vi "constructor.vi"(8 "error in (no error)":errorcluster, 9 "deviceDataBase":refnum<class "deviceDataBase.lvclass">, 10 "Path":path, 11 "compiledTime":timestamp) -> (0 "error out":errorcluster, 1 "error":bool, 2 "DeviceArray":refnum<class "DeviceArray.lvclass">, 3 "ScriptListCompiler out":refnum<class "ScriptListCompiler.lvclass">)   [LabVIEW 2009, in "Compiler.lvlib" / "ScriptListCompiler.lvclass"]
uses:
  ScriptListCompiler.lvclass
  DatabaseHelpers/DbConnection/DeviceDataBase/deviceDataBase.lvclass
  DatabaseHelpers/Database Objects/DeviceArray/DeviceArray.lvclass
  Scripting/DataPointScript/DataPointScript.lvclass
  ScriptListCompiler.lvclass/ScriptListCompiler.ctl
  Scripting/ScriptingEvent/ScriptEventList/ScriptEventList.lvclass
  Compiler.lvlib
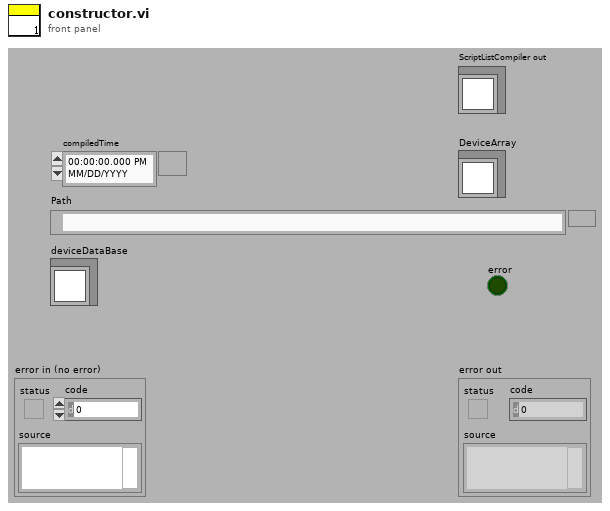
[diagram p1: front panel]
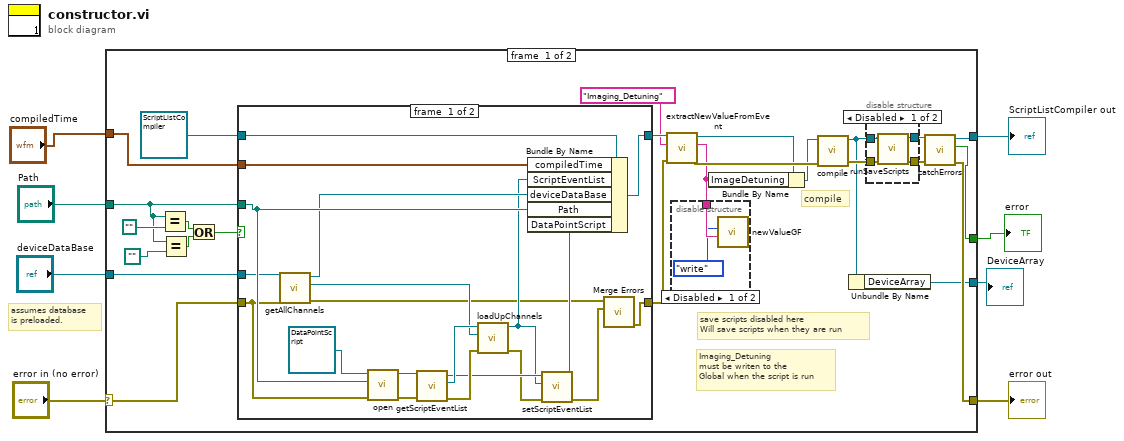
[diagram p0: block diagram]
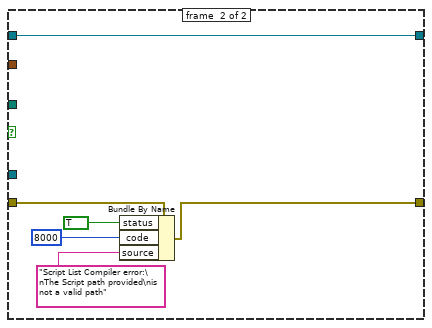
[diagram p4: hidden frame]
diagram:
  # "assumes database\nis preloaded."
  n1 = case shown="No Error" "error in (no error)" {
    selector: "error in (no error)" -> [w25 w68]
    tunnel: [w23 w68] -> w7
    tunnel: [w24 _] -> w4
    tunnel: "Path" -> [w26 _]
    tunnel: "deviceDataBase" -> [w29 _]
    tunnel: [w22 _] -> w3
    tunnel: "compiledTime" -> [w21 _]
    tunnel: [w20 _] -> w2
    frame #0 {
      # "Imaging_Detuning\nmust be writen to the\nGlobal when the script is run"
      # "save scripts disabled here\nWill save scripts when they are run"
      # "compile"
      n2 = Equal?(x=w26, y=path "") -> (x = y?=w32:bool)
      n3 = Equal?(x=w26, y=path "") -> (x = y?=w31:bool)
      n4 = Or(x=w32, y=w31) -> (x .or. y?=w28:bool)
      n5 = case shown="False" w28 {
        tunnel: w29 -> [w53 _]
        tunnel: refnum<class "ScriptListCompiler.lvclass"> refnum ("SettingsProcessors.lvlib:ScriptListCompiler.lvclass") -> [w61 w62]
        tunnel: [w60 w62] -> w19
        tunnel: w26 -> [w54 _]
        tunnel: w25 -> [w51 w67]
        tunnel: [w45 w66] -> w17
        tunnel: w21 -> [w42 _]
        frame #0 {
          n6 = call "getAllChannels.vi"("error in (no error)"=w51, "deviceDataBase in"=w53) -> ("error out"=w44:errorcluster, "ChannelArray.lvclass"=w50:refnum<class "ChannelArray.lvclass">, "deviceDataBase out"=w52:refnum<class "deviceDataBase.lvclass">)  [unwired: 7 in]
          n7 = call "open.vi"("error in (no error)"=w51, "Path"=w54, "DataPointScript in"=refnum<class "DataPointScript.lvclass"> refnum ("Tools.lvlib:Scripting.lvlib:DataPointScript.lvclass")) -> ("error out"=w57:errorcluster, "DataPointScript out"=w58:refnum<class "DataPointScript.lvclass">)  [unwired: 7 in]
          n8 = call "getScriptEventList.vi"("error in (no error)"=w57, "DataPointScript.lvclass in"=w58) -> ("error out"=w55:errorcluster, "ScriptEventList"=w56:refnum<class "ScriptEventList.lvclass">, "DataPointScript.lvclass out"=w49:refnum<class "DataPointScript.lvclass">)  [unwired: 7 in]
          n9 = call "loadUpChannels.vi"("error in (no error)"=w55, "ChannelArray"=w50, "ScriptEventList in"=w56) -> ("error out"=w48:errorcluster, "ScriptEventList out"=w47:refnum<class "ScriptEventList.lvclass">)  [unwired: 7 in]
          n10 = call "setScriptEventList.vi"("error in (no error)"=w48, "TScriptEventList"=w47, "DataPointScript.lvclass in"=w49) -> ("error out"=w43:errorcluster, "DataPointScript.lvclass out"=w46:refnum<class "DataPointScript.lvclass">)  [unwired: 7 in]
          n11 = Bundle By Name(cluster=w61, "compiledTime"=w42, "ScriptEventList"=w47, "deviceDataBase"=w52, "Path"=w54, "DataPointScript"=w46) -> (w60:refnum<class "ScriptListCompiler.lvclass">)
          n12 = call <vilib>:"Merge Errors.vi"("error in 2 (no error)"=w43, "error in 1 (no error)"=w44) -> ("error out"=w45:errorcluster)  [unwired: 5 in]
        }
        frame #1 {
          n13 = Bundle By Name(cluster=w67, "status"=TRUE, "code"=8000, "source"="Script List Compiler error:\nThe Script path provided\nis not a valid path") -> (w66:errorcluster)
        }
      }
      n14 = call "extractNewValueFromEvent.vi"("error in (no error)"=w17, "channelName"="Imaging_Detuning", "ScriptListCompiler in"=w19) -> ("error out"=w18:errorcluster, "newValue"=w9:string, "ScriptListCompiler out"=w11:refnum<class "ScriptListCompiler.lvclass">)  [unwired: 6 in]
      n15 = disable-structure shown="Disabled" {
        disable-tunnel: w9 -> [w35 _]
        frame #0 {
          n16 = call "newValueGF.vi"("newValue"=w35, "control"=enum16{"read", "write"}."write") -> ()  [unwired: 9 in, 1 out]
        }
        frame #1 {
        }
      }
      n17 = Bundle By Name(cluster=w11, "ImageDetuning"=w9) -> (w10:refnum<class "ScriptListCompiler.lvclass">)
      n18 = call-dynamic "compile.vi"("error in (no error)"=w18, "ScriptListCompiler in"=w10) -> ("error out"=w14:errorcluster, "ScriptListCompiler out"=w13:refnum<class "ScriptListCompiler.lvclass">)  [unwired: 8 in]
      n19 = Unbundle By Name(w13) -> ("DeviceArray"=w20:refnum<class "DeviceArray.lvclass">)
      n20 = disable-structure shown="Disabled" {
        disable-tunnel: [w39 w40] -> w15
        disable-tunnel: w14 -> [w38 w40]
        disable-tunnel: w13 -> [w37 w41]
        disable-tunnel: [w36 w41] -> w12
        frame #0 {
          n21 = call "runSaveScripts.vi"("error in (no error)"=w38, "ScriptListCompiler in"=w37) -> ("error out"=w39:errorcluster, "ScriptListCompiler out"=w36:refnum<class "ScriptListCompiler.lvclass">)  [unwired: 8 in]
        }
        frame #1 {
        }
      }
      n22 = call "catchErrors.vi"("error in (no error)"=w15, "ScriptListCompiler in"=w12) -> ("error out"=w23:errorcluster, "error"=w22:bool, "ScriptListCompiler out"=w24:refnum<class "ScriptListCompiler.lvclass">)  [unwired: 7 in]
    }
    frame #1 {
    }
  }
  "error out" <- w7
  "ScriptListCompiler out" <- w4
  "error" <- w3
  "DeviceArray" <- w2
